vi "Pendulum get Tx Latency ms.vi"(11 "instance":i32) -> (3 "function return":dbl)   [LabVIEW 2025, in "pendulumApp.lvlib"]
doc: "OOTB_API double Pendulum_getTxLatency_ms(int instance);"
uses:
  pendulumApp.lvlib
  pendulumApp.dll
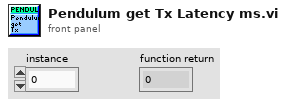
[diagram p1: front panel]
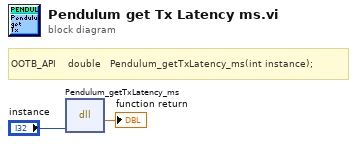
[diagram p0: block diagram]
diagram:
  # "OOTB_API    double   Pendulum_getTxLatency_ms(int instance);"
  n1 = dll-call lib="C:/Users/noaht/School/Fall 2025/Controls Lab/Lab 3/FA25_pend_Lab3_4/SADI_Pendulum_lib/pendulumApp.*" fn="Pendulum_getTxLatency_ms"("instance"="instance") -> (→"function return":dbl)  [unwired: 4 in, 2 out]
